vi "CLI_DeleteParam.vi"(8 "error in (no error)":errorcluster caption="entrée d'erreur (pas d'erreur)", 10 "ParsedParametersIn":cluster{"Name":string, "Value":string}[](array[cluster]), 11 "ParamToDelete":string) -> (0 "Error out":errorcluster, 2 "ParsedParametersOut":cluster{"Name":string, "Value":string}[](array[cluster]), 3 "Deleted":bool)   [LabVIEW 2013]
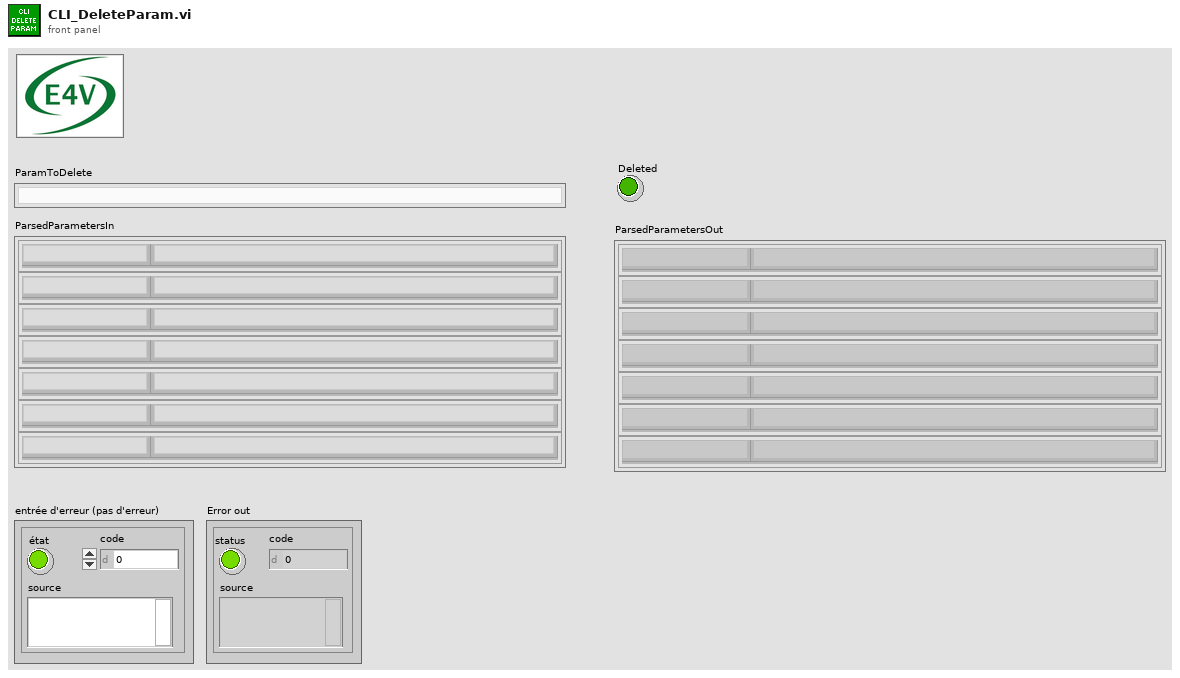
[diagram p1: front panel]
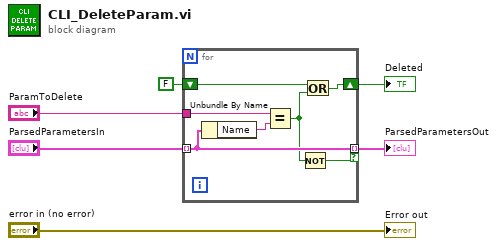
[diagram p0: block diagram]
diagram:
  n1 = for {
    tunnel: "ParsedParametersIn" -> [w11] mode=indexing
    tunnel: "ParamToDelete" -> [w13]
    shift-right: [w9] -> w3
    shift-left: FALSE -> [w10]
    tunnel: [w11] -> w1 mode=indexing if=w8
    n2 = Unbundle By Name(w11) -> ("Name"=w12:string)
    n3 = Equal?(x=w13, y=w12) -> (x = y?=w7:bool)
    n4 = Not(x=w7) -> (.not. x?=w8:bool)
    n5 = Or(x=w10, y=w7) -> (x .or. y?=w9:bool)
  }
  "Deleted" <- w3
  "ParsedParametersOut" <- w1
  "Error out" <- "error in (no error)"
